vi "Custom Serial Number Dialog.vi"(9 "Automated":bool, 11 "Sequence Context In":refnum<k7>) -> (0 "error out":errorcluster, 2 "Serial":string, 3 "Continue Testing":bool)   [LabVIEW 2025]
uses:
  <vilib>/addons/TestStand/_TSUtility.llb/TestStand - Get Property Value (Boolean).vi
  <vilib>/addons/TestStand/_TSUtility.llb/TestStand - Get Property Value (String).vi
  <vilib>/addons/TestStand/_TSUtility.llb/TestStand - Start Modal Dialog (Sequence Context).vi
  <vilib>/addons/TestStand/_TSUtility.llb/TestStand - End Modal Dialog (Sequence Context).vi
  <vilib>/addons/TestStand/_TSUtility.llb/TestStand - Get Property Value (Number {Signed 32-bit Integer}).vi
  Program Files (x86)/National Instruments/LabVIEW 2024/Instr.lib/Driver Simulation/Fixture.lvlib
panel:
  in  "stop":bool
  in  "OK":bool
  in  "UUT Serial Number":u16(ring) items=["0", "1", "2", "3", "4", "5", "6", "7", "8", "9", "AllFail", "Fail", "Golden", "Pass", "ResistanceFail", "ThermalFail"]
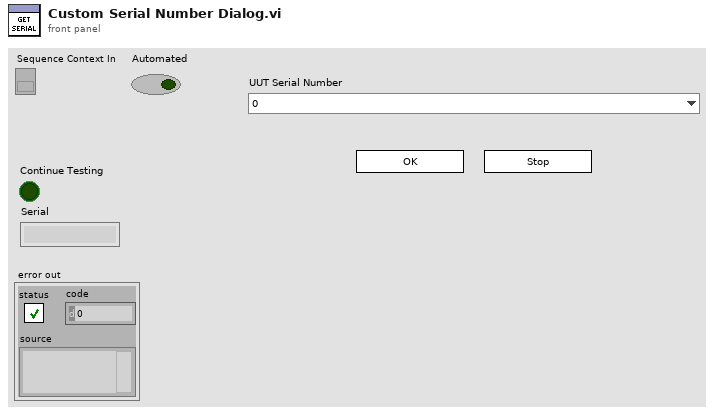
[diagram p1: front panel]
types:
  T1 = enum32{"Invalid", "Standard", "Closed", "Hidden", "Minimized", "Maximized"}
  T2 = typedef "TestStand - Status Monitor.ctl" = cluster{"Sequence Context":refnum<k7>, "Execution":refnum<k7>, "Termination Monitor":refnum<k7>}
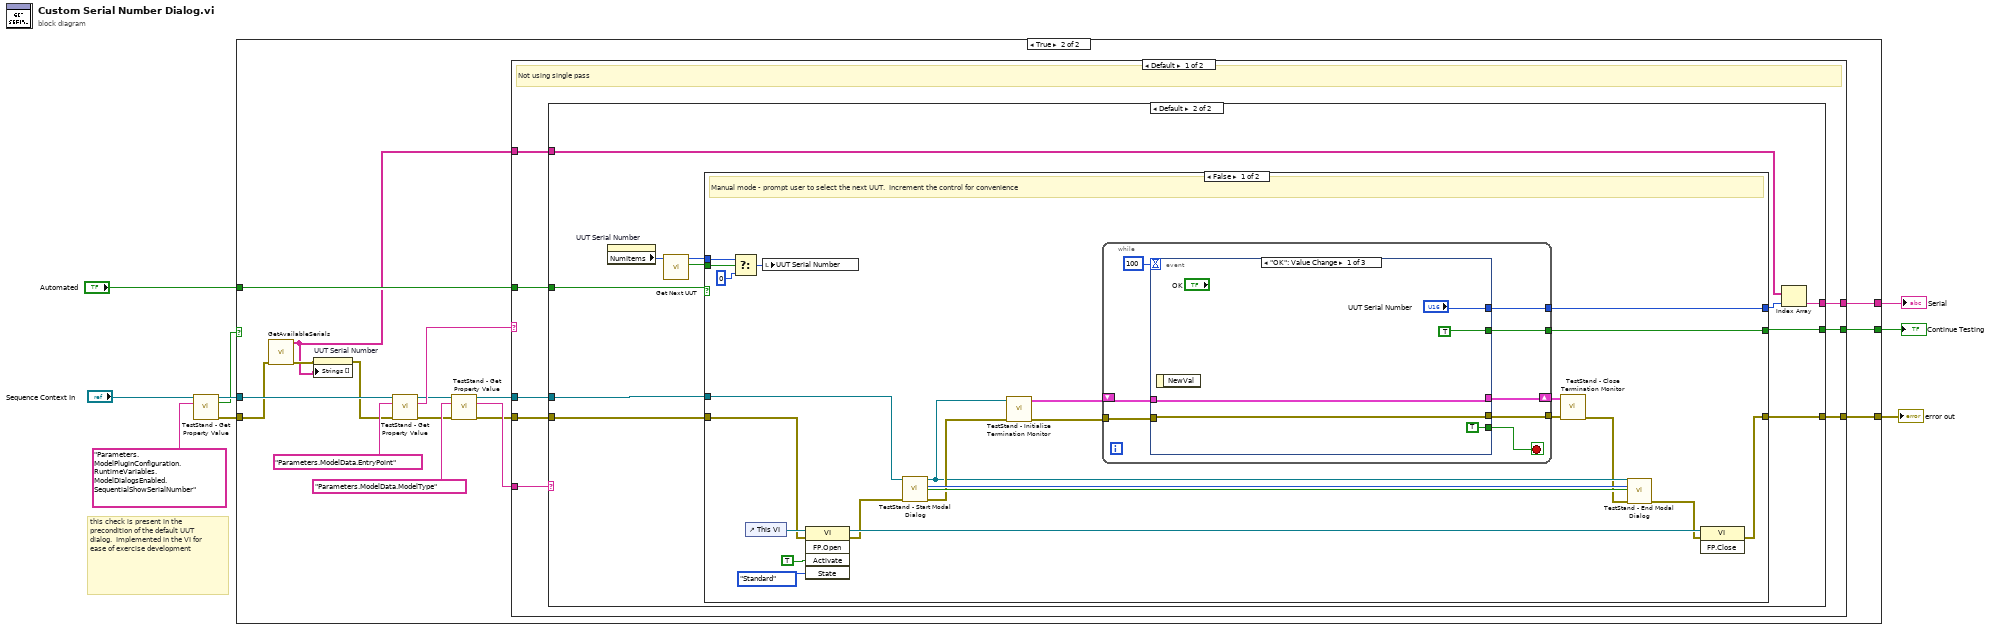
[diagram p0: block diagram]
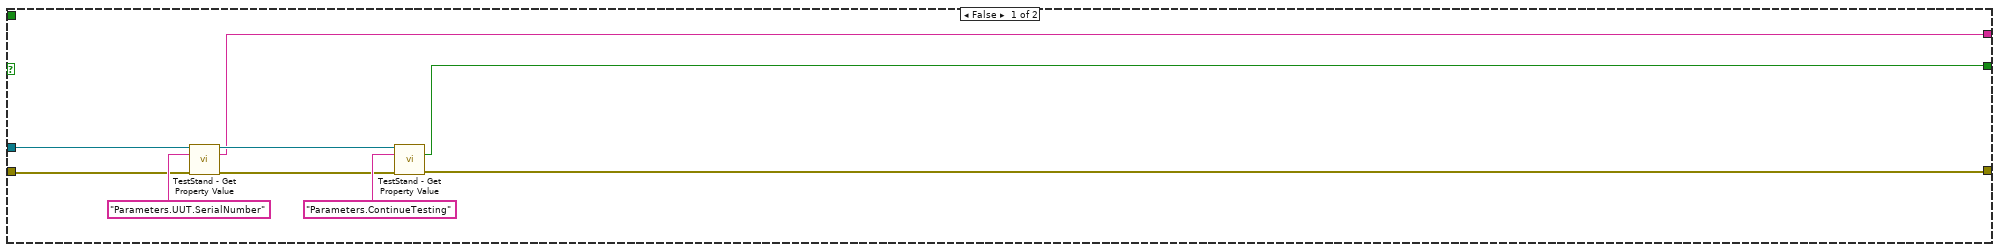
[diagram p2: hidden frame]
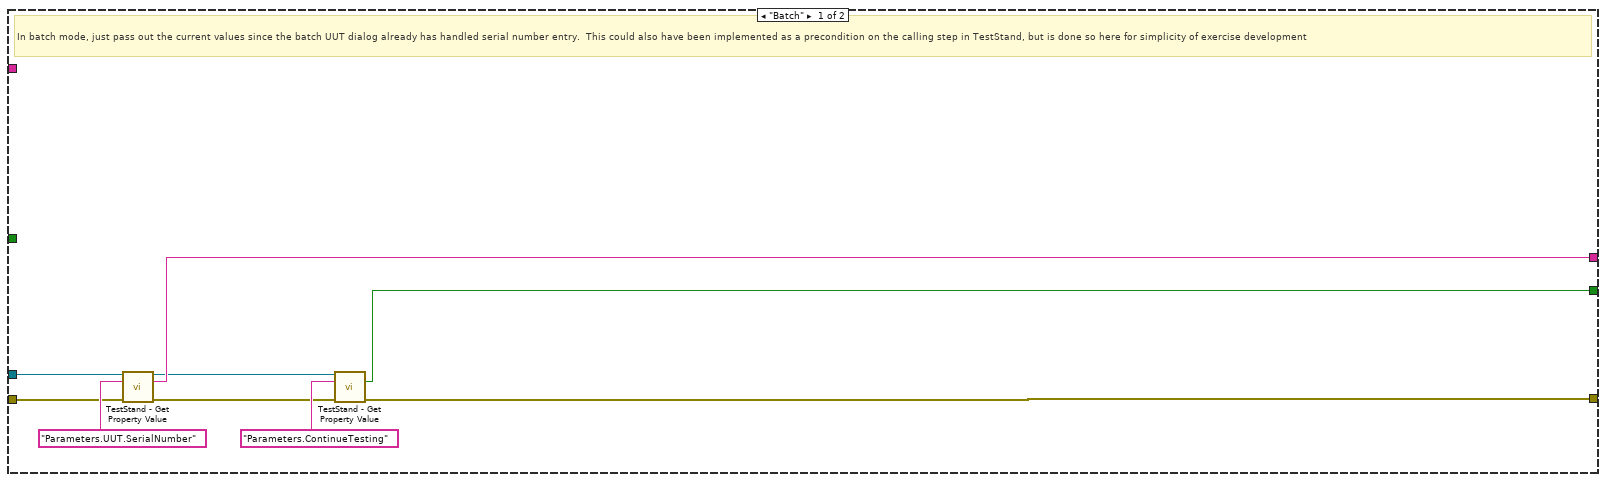
[diagram p3: hidden frame]
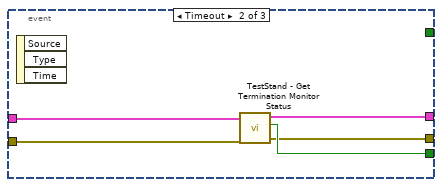
[diagram p4: hidden frame]
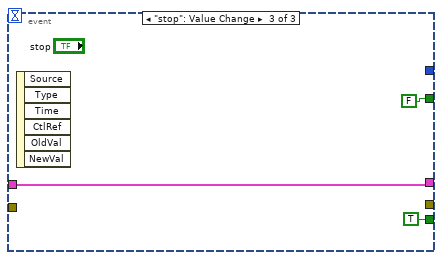
[diagram p5: hidden frame]
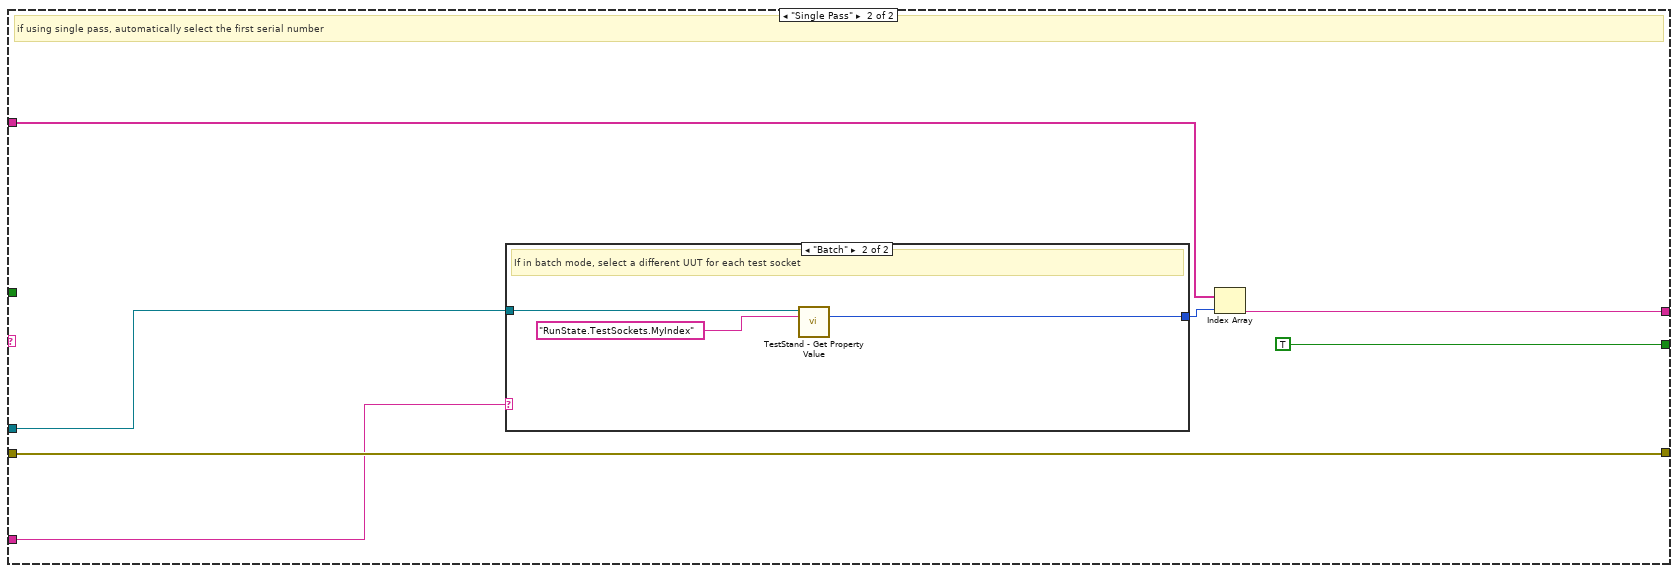
[diagram p7: hidden frame]
diagram:
  # "this check is present in the precondition of the default UUT dialog.  Implemented in the VI for ease of exercise development"
  n1 = call-poly <vilib>:"TestStand - Get Property Value.vi"("Sequence Context In"="Sequence Context In", "Lookup String"="Parameters.ModelPluginConfiguration.RuntimeVariables.ModelDialogsEnabled.SequentialShowSerialNumber") -> ("Sequence Context Out"=w5:refnum<k7>, "Value"=w1:bool, "error out"=w2:errorcluster)  [unwired: 11 in]
  n2 = case shown="True" w1 {
    tunnel: [w11 w35] -> w9
    tunnel: "Automated" -> [_ w31]
    tunnel: [w10 w30] -> w7
    tunnel: [w12 w24] -> w6
    tunnel: w5 -> [w13 w21]
    tunnel: w2 -> [w14 w20]
    frame False {
      n3 = call-poly <vilib>:"TestStand - Get Property Value.vi"("Sequence Context In"=w13, "Lookup String"="Parameters.UUT.SerialNumber", "error in (no error)"=w14) -> ("Sequence Context Out"=w16:refnum<k7>, "Value"=w12:string, "error out"=w15:errorcluster)  [unwired: 10 in]
      n4 = call-poly <vilib>:"TestStand - Get Property Value.vi"("Sequence Context In"=w16, "Lookup String"="Parameters.ContinueTesting", "error in (no error)"=w15) -> ("Value"=w11:bool, "error out"=w10:errorcluster)  [unwired: 10 in, 1 out]
    }
    frame True {
      n5 = call "GetAvailableSerials.vi"("error in (no error)"=w20) -> ("error out"=w32:errorcluster, "serialNumbers"=w25:string[])  [unwired: 9 in]
      n6 = property on="UUT Serial Number" class="Ring (strict)"(error in=w32, "Strings []"=w25) -> (error out=w19:errorcluster)  [unwired: 1 in, 1 out]
      n7 = call-poly <vilib>:"TestStand - Get Property Value.vi"("Sequence Context In"=w21, "Lookup String"="Parameters.ModelData.EntryPoint", "error in (no error)"=w19) -> ("Sequence Context Out"=w28:refnum<k7>, "Value"=w33:string, "error out"=w23:errorcluster)  [unwired: 10 in]
      n8 = call-poly <vilib>:"TestStand - Get Property Value.vi"("Sequence Context In"=w28, "Lookup String"="Parameters.ModelData.ModelType", "error in (no error)"=w23) -> ("Sequence Context Out"=w27:refnum<k7>, "Value"=w26:string, "error out"=w22:errorcluster)  [unwired: 10 in]
      n9 = case shown="Default" w33 {
        tunnel: [w43 w112] -> w24
        tunnel: [w42 TRUE] -> w35
        tunnel: [w41 w117] -> w30
        tunnel: w31 -> [w40 _]
        tunnel: w27 -> [w39 w116]
        tunnel: w22 -> [w38 w117]
        tunnel: w26 -> [w37 w115]
        tunnel: w25 -> [w36 w113]
        frame Default {
          # "Not using single pass"
          n10 = case shown="Default" w37 {
            tunnel: [w48 w53] -> w43
            tunnel: [w49 w63] -> w42
            tunnel: [w46 w62] -> w41
            tunnel: w40 -> [_ w61]
            tunnel: w39 -> [w52 w60]
            tunnel: w38 -> [w44 w59]
            tunnel: w36 -> [_ w54]
            frame "Batch" {
              # "In batch mode, just pass out the current values since the batch UUT dialog already has handled serial number entry.  This could also have been implemented as a precondition on the calling step in TestStand, but is done so here for simplicity of exercise development"
              n11 = call-poly <vilib>:"TestStand - Get Property Value.vi"("Sequence Context In"=w52, "Lookup String"="Parameters.UUT.SerialNumber", "error in (no error)"=w44) -> ("Sequence Context Out"=w47:refnum<k7>, "Value"=w48:string, "error out"=w45:errorcluster)  [unwired: 10 in]
              n12 = call-poly <vilib>:"TestStand - Get Property Value.vi"("Sequence Context In"=w47, "Lookup String"="Parameters.ContinueTesting", "error in (no error)"=w45) -> ("Value"=w49:bool, "error out"=w46:errorcluster)  [unwired: 10 in, 1 out]
            }
            frame Default {
              n13 = property on="UUT Serial Number" class="Ring (strict)"() -> ("NumItems"=w58:u32)  [unwired: 2 in, 2 out]
              n14 = call "Get Next UUT.vi"("Number of UUTs"=w58) -> ("End of List"=w57:bool, "next UUT"=w56:u16)  [unwired: 9 in]
              n15 = case shown="False" w61 {
                tunnel: [w87 w109] -> w55
                tunnel: [w86 w110] -> w63
                tunnel: [w83 w111] -> w62
                tunnel: w60 -> [w80 _]
                tunnel: w59 -> [w75 w111]
                tunnel: w57 -> [w74 w110]
                tunnel: w56 -> [w71 w109]
                frame False {
                  # "Manual mode - prompt user to select the next UUT.  Increment the control for convenience"
                  n16 = Select(t=w71, s=w74, f=u16 0) -> (s? t:f=w72:u16)
                  n17 = control-ref of="This VI"() -> (w76:refnum<vi>)
                  n18 = local write "UUT Serial Number"(w72) -> ()
                  n19 = invoke class="VI" method="FP.Open"(reference=w76, error in=w75, "Activate"=TRUE ("Activate?"), "State"=T1."Standard") -> (reference out=w82:refnum<vi>, error out=w79:errorcluster)  [unwired: 1 in, 3 out]
                  n20 = call-poly <vilib>:"TestStand - Start Modal Dialog.vi"("Sequence Context In"=w80, "error in (no error)"=w79) -> ("Sequence Context Out"=w69:refnum<k7>, "Modal ID"=w78:i32, "VI Originally Open"=w77:bool, "error out"=w70:errorcluster)  [unwired: 9 in, 1 out]
                  n21 = call <vilib>:"TestStand - Initialize Termination Monitor.vi"("error in (no error)"=w70, "Sequence Context In"=w69) -> ("error out"=w68:errorcluster, "Status Monitor Out"=w67:T2)  [unwired: 8 in]
                  n22 = while {
                    tunnel: [w95] -> w87
                    tunnel: [w94] -> w86
                    tunnel: w68 -> [w93]
                    tunnel: [w92] -> w66
                    shift-right: [w88] -> w65
                    shift-left: w67 -> [w90]
                    stop <- w91 stop-if-true
                    n23 = event shown="[0] \"OK\": Value Change" {
                      selector: _ -> [_ _ _]
                      dyn-events: _ -> [_ _ _]
                      timeout: 100 -> [_ _ _]
                      tunnel: ["UUT Serial Number" _ _] -> w95
                      tunnel: [TRUE _ FALSE] -> w94
                      tunnel: [TRUE w103 TRUE] -> w91
                      tunnel: w93 -> [w97 w104 _]
                      tunnel: [w97 w102 _] -> w92
                      tunnel: w90 -> [w96 w105 w106]
                      tunnel: [w96 w101 w106] -> w88
                      event "OK": Value Change {
                        n24 = event-data() -> ()  [unwired: 1 in, 1 out]
                      }
                      event Timeout {
                        n25 = event-data() -> ()  [unwired: 1 in, 3 out]
                        n26 = call <vilib>:"TestStand - Get Termination Monitor Status.vi"("error in (no error)"=w104, "Status Monitor In"=w105) -> ("error out"=w102:errorcluster, "Terminating or Aborting"=w103:bool, "Status Monitor Out"=w101:T2)  [unwired: 7 in]
                      }
                      event "stop": Value Change {
                        n27 = event-data() -> ()  [unwired: 1 in, 6 out]
                      }
                    }
                  }
                  n28 = call <vilib>:"TestStand - Close Termination Monitor.vi"("error in (no error)"=w66, "Status Monitor In"=w65) -> ("error out"=w64:errorcluster)  [unwired: 9 in]
                  n29 = call-poly <vilib>:"TestStand - End Modal Dialog.vi"("Sequence Context In"=w69, "Modal ID"=w78, "VI Originally Open"=w77, "error in (no error)"=w64) -> ("error out"=w81:errorcluster)  [unwired: 11 in]
                  n30 = invoke class="VI" method="FP.Close"(reference=w82, error in=w81) -> (error out=w83:errorcluster)  [unwired: 1 in, 2 out]
                }
                frame True {
                  # "automation mode - select the next UUT"
                }
              }
              n31 = Index Array(array=w54, index=w55) -> (element=w53:string)
            }
          }
        }
        frame "Single Pass" {
          # "if using single pass, automatically select the first serial number"
          n32 = case shown="\"Batch\"" w115 {
            tunnel: w116 -> [_ w121]
            tunnel: [_ w119] -> w114
            frame Default {
            }
            frame "Batch" {
              # "If in batch mode, select a different UUT for each test socket"
              n33 = call-poly <vilib>:"TestStand - Get Property Value.vi"("Sequence Context In"=w121, "Lookup String"="RunState.TestSockets.MyIndex") -> ("Value"=w119:i32)  [unwired: 11 in, 2 out]
            }
          }
          n34 = Index Array(array=w113, index=w114) -> (element=w112:string)
        }
      }
    }
  }
  "Continue Testing" <- w9
  "Serial" <- w6
  "error out" <- w7
